vi "Test Indent.vi"() -> ()   [LabVIEW 2012]
doc: "SciScan 1.2 160622"
panel:
  out "All Decendants":string[](array[string])
  in  "Tree":string(tree)
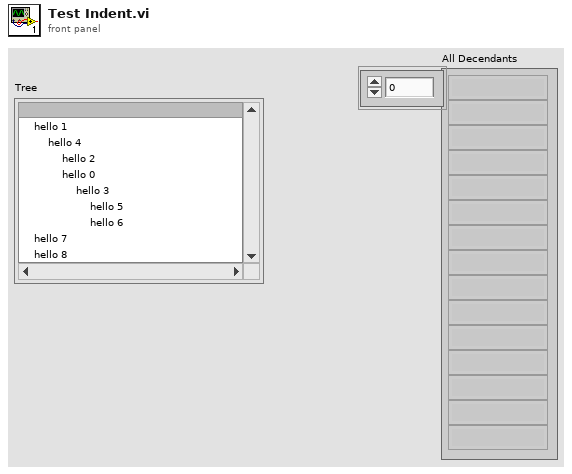
[diagram p1: front panel]
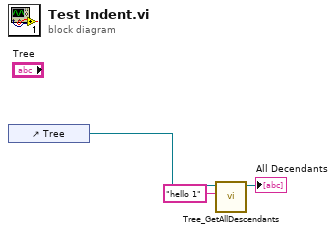
[diagram p0: block diagram]
diagram:
  n1 = control-ref of="Tree"() -> (w3:refnum<vi>)
  n2 = call "Tree_GetAllDescendants.vi"("Tag"="hello 1", "Tree Refnum IN"=w3) -> ("Tree Refnum OUT"=→"All Decendants":refnum<vi>)  [unwired: 7 in, 2 out]
